vi "Begin.vi"(8 "error in":errorcluster) -> (0 "error out":errorcluster)   [LabVIEW 2018]
doc: "Called before other user functions, this VI is expected to open initial I/O refnums, load in file data, and do all program initialization. Notice that the <B>error out</B> terminal is simply used for data flow. Wiring it to other structures or subVIs ensures that this VI runs first."
uses:
  <vilib>/Rock Robotics/WPI/DriverStation/WPI_DriverStationRobotMode2.ctl
  <vilib>/Rock Robotics/SystemInterfaces/DIO/FPGA_DIOPWMChannel.ctl
  <vilib>/Rock Robotics/WPI/Joystick/WPI_JoystickDeviceEnum.ctl
  <vilib>/Rock Robotics/SystemInterfaces/AI/FPGA_AIChannel.ctl
  Robot Global Data.vi
  <vilib>/Rock Robotics/WPI/RobotDrive/WPI_RobotDriveOpen4MotorWithTalon.vi
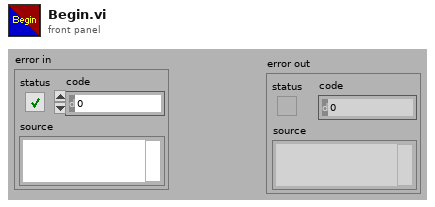
[diagram p1: front panel]
types:
  T1 = typedef "FPGA_AIChannel.ctl" = enum8{"AI 0", "AI 1", "AI 2", "AI 3", "AI MXP 0", "AI MXP 1", "AI MXP 2", "AI MXP 3", "Invalid"}
  T2 = typedef "WPI_JoystickDeviceEnum.ctl" = enum16{"USB 0", "USB 1", "USB 2", "USB 3", "USB 4", "USB 5"}
  T3 = typedef "FPGA_DIOPWMChannel.ctl" = enum8{"PWM 0", "PWM 1", "PWM 2", "PWM 3", "PWM 4", "PWM 5", "PWM 6", "PWM 7", "PWM 8", "PWM 9", "PWM MXP 0", "PWM MXP 1", "PWM MXP 2", "PWM MXP 3", "PWM MXP 4", "PWM MXP 5", "PWM MXP 6", "PWM MXP 7", "PWM MXP 8", "PWM MXP 9", "Invalid"}
  T4 = typedef "WPI_DriverStationRobotMode2.ctl" = enum16{"Autonomous Disabled", "Autonomous Enabled", "Teleop Disabled", "Teleop Enabled", "Disconnected", "Finish", "Test Disabled", "Test Enabled", "Emergency Stopped"}
  T5 = typedef "WPI_RobotDriveDevRef.ctl" = cluster{"DevStatus":errorcluster, "Motors[]":T6[], "Square Inputs":bool, "Max Output":dbl}
  T6 = typedef "WPI_MotorControlDeviceRef.ctl" = cluster{"DeviceStatus":errorcluster, "Type":T7, "PWM":cluster{"PWM Channel":T3, "DeadBand":T8}, "CAN":cluster{"Device Number":u8, "SetOutput VI Ref":variant, "GetOutput VI Ref":variant, "Enable VI Ref":variant, "Disable VI Ref":variant, "Data":variant}, "Invert":bool, "DIO PWM":cluster{"PWM \"Enable\" Channel":T3, "DIOChannel":T9, "PWM Rate":dbl}}
  T7 = typedef "WPI_MotorControlType.ctl" = enum16{"PWM", "CAN", "DIO PWM"}
  T8 = typedef "WPI_PWMDeadband.ctl" = cluster{"Name":string, "maxPositivePwm":i32, "minPositivePwm":i32, "centerPwm":i32, "maxNegativePwm":i32, "minNegativePwm":i32, "angularRange":u16}
  T9 = typedef "FPGA_DIOChannel.ctl" = enum8{"DIO 0", "DIO 1", "DIO 2", "DIO 3", "DIO 4", "DIO 5", "DIO 6", "DIO 7", "DIO 8", "DIO 9", "DIO MXP 0", "DIO MXP 1", "DIO MXP 2", "DIO MXP 3", "DIO MXP 4", "DIO MXP 5", "DIO MXP 6", "DIO MXP 7", "DIO MXP 8", "DIO MXP 9", "DIO MXP 10", "DIO MXP 11", "DIO MXP 12", "DIO MXP 13", "DIO MXP 14", "DIO MXP 15", "SPI Port CS1", "SPI Port CS2", "SPI Port CS3", "SPI Port MISO", "SPI Port MOSI", "Invalid"}
  T10 = typedef "WPI_JoystickDevRef.ctl" = cluster{"Device":T2}
  T11 = typedef "WPI_AnalogChannelDevRef.ctl" = cluster{"DevStatus":errorcluster, "Analog Channel":T1}
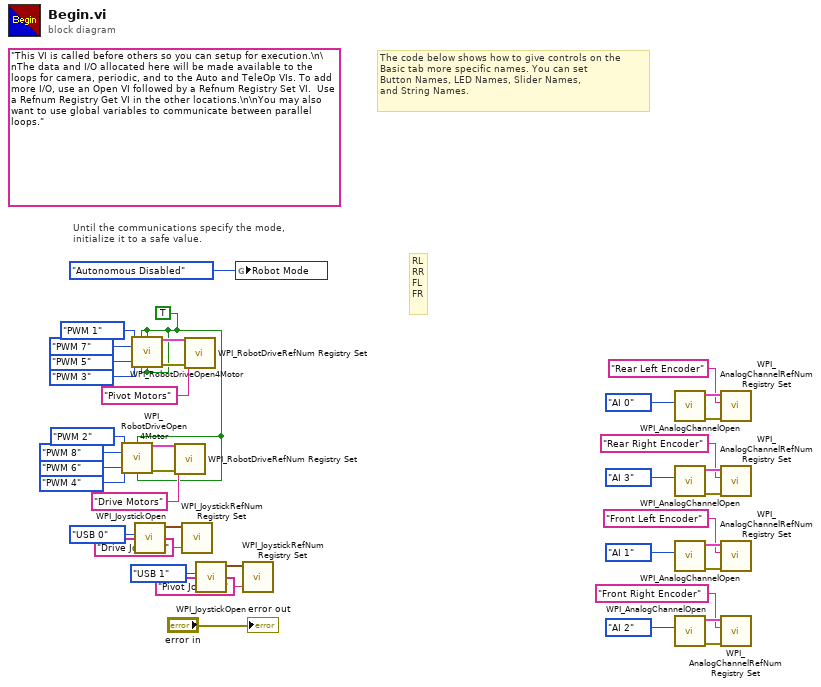
[diagram p0: block diagram]
diagram:
  w1 = TRUE
  (unwired) "This VI is called before others so you can setup for execution.\n\nThe data and I/O allocated here will be made available to the loops for camera, periodic, and to the Auto and TeleOp VIs. To add more I/O, use an Open VI followed by a Refnum Registry Set VI.  Use a Refnum Registry Get VI in the other locations.\n\nYou may also want to use global variables to communicate between parallel loops."
  # "RL\nRR\nFL\nFR"
  # "The code below shows how to give controls on the\nBasic tab more specific names. You can set\nButton Names, LED Names, Slider Names,\nand String Names."
  # "Until the communications specify the mode,\ninitialize it to a safe value."
  n1 = call-poly <vilib>:"WPI_RobotDriveOpen4Motor.vi"("Rear Left Motor"=FPGA_DIOPWMChannel."PWM 2", "Rear Right Motor Inverted"=w1, "Rear Right Motor"=FPGA_DIOPWMChannel."PWM 8", "Front Left Motor"=FPGA_DIOPWMChannel."PWM 6", "Front Right Motor"=FPGA_DIOPWMChannel."PWM 4", "Front Right Motor Inverted"=w1) -> ("RobotDriveDevRef"=w25:T5, "error out"=w26:errorcluster)  [unwired: 8 in]
  n2 = call-poly <vilib>:"WPI_RobotDriveOpen4Motor.vi"("Rear Left Motor"=FPGA_DIOPWMChannel."PWM 1", "Rear Left Motor Inverted"=w1, "Rear Right Motor Inverted"=w1, "Rear Right Motor"=FPGA_DIOPWMChannel."PWM 7", "Front Left Motor"=FPGA_DIOPWMChannel."PWM 5", "Front Right Motor"=FPGA_DIOPWMChannel."PWM 3", "Front Left Motor Inverted"=w1, "Front Right Motor Inverted"=w1) -> ("RobotDriveDevRef"=w32:T5, "error out"=w33:errorcluster)  [unwired: 6 in]
  n3 = call <vilib>:"WPI_JoystickOpen.vi"("JoystickDevice"=WPI_JoystickDeviceEnum."USB 0") -> ("JoystickDevRef"=w22:T10)  [unwired: 10 in]
  n4 = call <vilib>:"WPI_RobotDriveRefNum Registry Set.vi"("error in (no error)"=w26, "refnum name"="Drive Motors", "RobotDriveDevRef"=w25) -> ()  [unwired: 7 in, 2 out]
  n5 = call <vilib>:"WPI_JoystickRefNum Registry Set.vi"("refnum name"="Drive Joystick", "JoystickDevRef"=w22) -> ()  [unwired: 8 in, 2 out]
  n6 = call <vilib>:"WPI_RobotDriveRefNum Registry Set.vi"("error in (no error)"=w33, "refnum name"="Pivot Motors", "RobotDriveDevRef"=w32) -> ()  [unwired: 7 in, 2 out]
  n7 = call <vilib>:"WPI_JoystickOpen.vi"("JoystickDevice"=WPI_JoystickDeviceEnum."USB 1") -> ("JoystickDevRef"=w19:T10)  [unwired: 10 in]
  n8 = global write "Robot Global Data.vi" "Robot Mode"(WPI_DriverStationRobotMode2."Autonomous Disabled" ("Robot Mode")) -> ()
  n9 = call <vilib>:"WPI_JoystickRefNum Registry Set.vi"("refnum name"="Pivot Joystick", "JoystickDevRef"=w19) -> ()  [unwired: 8 in, 2 out]
  n10 = call <vilib>:"WPI_AnalogChannelOpen.vi"("Analog Channel"=FPGA_AIChannel."AI 0") -> ("error out"=w5:errorcluster, "AIDeviceRef"=w4:T11)  [unwired: 9 in]
  n11 = call <vilib>:"WPI_AnalogChannelOpen.vi"("Analog Channel"=FPGA_AIChannel."AI 3") -> ("error out"=w9:errorcluster, "AIDeviceRef"=w8:T11)  [unwired: 9 in]
  n12 = call <vilib>:"WPI_AnalogChannelOpen.vi"("Analog Channel"=FPGA_AIChannel."AI 1") -> ("error out"=w13:errorcluster, "AIDeviceRef"=w12:T11)  [unwired: 9 in]
  n13 = call <vilib>:"WPI_AnalogChannelOpen.vi"("Analog Channel"=FPGA_AIChannel."AI 2") -> ("error out"=w17:errorcluster, "AIDeviceRef"=w16:T11)  [unwired: 9 in]
  n14 = call <vilib>:"WPI_AnalogChannelRefNum Registry Set.vi"("error in (no error)"=w5, "refnum name"="Rear Left Encoder", "AIDeviceRef"=w4) -> ()  [unwired: 7 in, 2 out]
  n15 = call <vilib>:"WPI_AnalogChannelRefNum Registry Set.vi"("error in (no error)"=w9, "refnum name"="Rear Right Encoder", "AIDeviceRef"=w8) -> ()  [unwired: 7 in, 2 out]
  n16 = call <vilib>:"WPI_AnalogChannelRefNum Registry Set.vi"("error in (no error)"=w13, "refnum name"="Front Left Encoder", "AIDeviceRef"=w12) -> ()  [unwired: 7 in, 2 out]
  n17 = call <vilib>:"WPI_AnalogChannelRefNum Registry Set.vi"("error in (no error)"=w17, "refnum name"="Front Right Encoder", "AIDeviceRef"=w16) -> ()  [unwired: 7 in, 2 out]
  "error out" <- "error in"
